vi "McP_Step-WL_Converter.vi"(0 "Wavelength Unit":T2=enum."nm", 1 "Option (Z0 <=> WL)":enum16{"Z0 => WL", "WL => Z0", "Update WL only"}(ring), 5 "Grating Density":T1=enum."1200", 7 "Velocity (Steps/s)":i32=42372, 9 "Stepper Position Input":i32 min=-8388607 max=8388607, 12 "Wavelength Input":dbl format="%.2f") -> (3 "Precision":i32, 4 "Wavelength Output":dbl format="%.2f", 6 "Current Couter Position":dbl format="%.2f", 8 "nm Output":dbl format="%.2f", 10 "Slew Rate":dbl format="%.2f", 13 "X-Axis Unit String":string, 14 "UnitFormatString":string="nm", 15 "Stepper Position Output":i32 min=-8388607 max=8388607)   [LabVIEW 2021]
doc: "(1) Convert stepper position to its corresponding wavelength (in the given unit and grating setting)\n(2) Vice versa."
uses:
  Globals and TypeDefs/Type Definitions.llb/Wavelength Unit.ctt
  Globals and TypeDefs/Type Definitions.llb/McPherson Grating Density.ctl
  Globals and TypeDefs/gSpectrometer.vi
  File and save/X-Axis Converter.llb/X-Point Converter.vi
  File and save/X-Axis Converter.llb/X-Axis Converter.vi
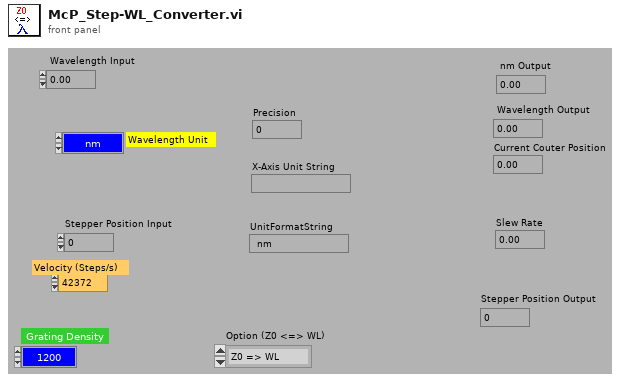
[diagram p1: front panel]
types:
  T1 = typedef "McPherson Grating Density.ctl" = enum8{"150", "300", "600", "1200", "1800"}
  T2 = typedef "Wavelength Unit.ctt" = enum8{"Point", "nm", "eV", "meV", "cm_1"}
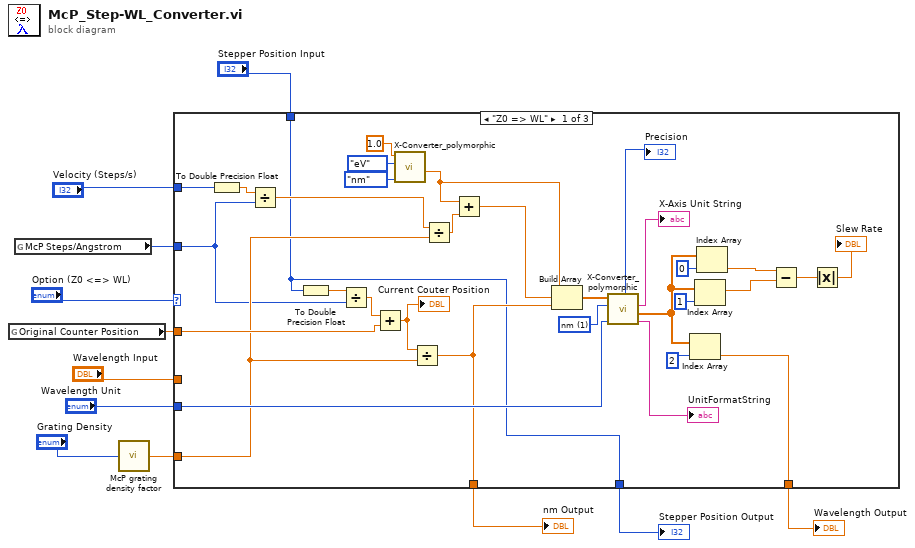
[diagram p0: block diagram]
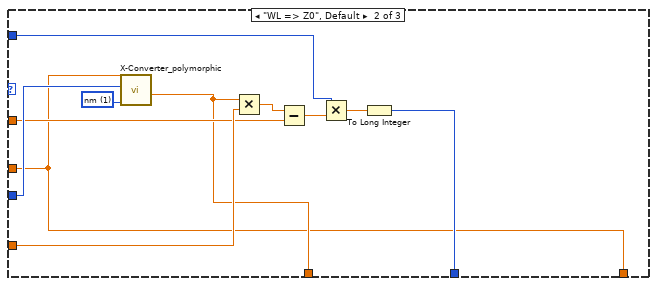
[diagram p2: hidden frame]
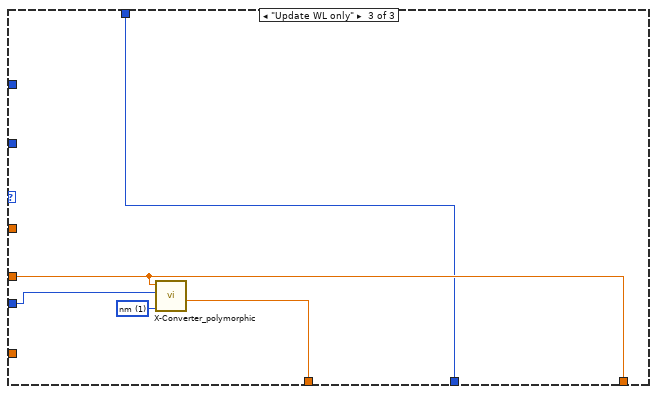
[diagram p3: hidden frame]
diagram:
  n1 = global read "gSpectrometer.vi" "Original Counter Position"() -> (w3:dbl)
  n2 = global read "gSpectrometer.vi" "McP Steps/Angstrom"() -> (w4:i32)
  n3 = call "McP grating density factor.vi"("Grating Density"="Grating Density") -> ("GratingFactor"=w5:dbl)
  n4 = case shown="\"Z0 => WL\"" "Option (Z0 <=> WL)" {
    tunnel: w3 -> [w28 w51 _]
    tunnel: w4 -> [w15 w50 _]
    tunnel: "Velocity (Steps/s)" -> [w17 _ _]
    tunnel: "Wavelength Unit" -> [w27 w55 w59]
    tunnel: w5 -> [w22 w53 _]
    tunnel: [w14 w47 w56] -> w12
    tunnel: [w26 w45 w57] -> w10
    tunnel: "Stepper Position Input" -> [w14 _ w56]
    tunnel: [w23 w46 w58] -> w9
    tunnel: "Wavelength Input" -> [_ w45 w57]
    frame "Z0 => WL" {
      w41 = 1 items=["Point #", "nm", "eV", "meV", "cm-1"] ("Old X-Axis Unit")
      n5 = To Double Precision Float(number=w17) -> (double precision float=w16:dbl)
      n6 = Divide(x=w16, y=w15) -> (x/y=w24:dbl)
      n7 = To Double Precision Float(number=w14) -> (double precision float=w13:dbl)
      n8 = Divide(x=w13, y=w15) -> (x/y=w44:dbl)
      n9 = Add(x=w44, y=w28) -> (x+y=w43:dbl)
      "Current Couter Position" <- w43
      n10 = call-poly "X-Converter_polymorphic.vi"("X-Axis Unit"=Wavelength_Unit.ctt."nm", "Old X-Axis Unit"=Wavelength_Unit.ctt."eV", "X-Axis input"=1.0 ("x")) -> ("X-Axis Output"=w19:dbl)  [unwired: 2 in, 3 out]
      n11 = Divide(x=w43, y=w22) -> (x/y=w23:dbl)
      n12 = Divide(x=w24, y=w22) -> (x/y=w25:dbl)
      n13 = Add(x=w19, y=w25) -> (x+y=w39:dbl)
      n14 = Build Array(w19, w39, w23) -> (w42:dbl[])
      n15 = call-poly "X-Converter_polymorphic.vi"("X-Axis Unit"=w27, "Old X-Axis Unit"=w41, "X-Axis input"=w42) -> ("UnitFormatString"=→"UnitFormatString":string, "X-Axis Output"=w38:dbl[], "X-Axis Unit String"=→"X-Axis Unit String":string, "Precision"=→"Precision":i32)  [unwired: 2 in]
      n16 = Index Array(array=w38, index=2 ("Index")) -> (element=w26:dbl)
      n17 = Index Array(array=w38, index=1 ("Index")) -> (element=w31:dbl)
      n18 = Index Array(array=w38, index=0 ("Index")) -> (element=w32:dbl)
      n19 = Subtract(x=w32, y=w31) -> (x-y=w34:dbl)
      n20 = Absolute Value(x=w34) -> (abs(x)=→"Slew Rate":dbl)
    }
    frame "WL => Z0", Default {
      w54 = 1 items=["Point #", "nm", "eV", "meV", "cm-1"] ("X-Axis Unit")
      n21 = call-poly "X-Converter_polymorphic.vi"("X-Axis Unit"=w54, "Old X-Axis Unit"=w55, "X-Axis input"=w45) -> ("X-Axis Output"=w46:dbl)  [unwired: 2 in, 3 out]
      n22 = Multiply(x=w46, y=w53) -> (x*y=w52:dbl)
      n23 = Subtract(x=w52, y=w51) -> (x-y=w49:dbl)
      n24 = Multiply(x=w50, y=w49) -> (x*y=w48:dbl)
      n25 = To Long Integer(number=w48) -> (32bit integer=w47:i32)
    }
    frame "Update WL only" {
      w60 = 1 items=["Point #", "nm", "eV", "meV", "cm-1"] ("X-Axis Unit")
      n26 = call-poly "X-Converter_polymorphic.vi"("X-Axis Unit"=w60, "Old X-Axis Unit"=w59, "X-Axis input"=w57) -> ("X-Axis Output"=w58:dbl)  [unwired: 2 in, 3 out]
    }
  }
  "Stepper Position Output" <- w12
  "Wavelength Output" <- w10
  "nm Output" <- w9
